vi "build waveform.vi"(10 "initialized array":dbl[][](array[numeric])) -> (2 "output waveform":waveform(dbl))   [LabVIEW 2014]
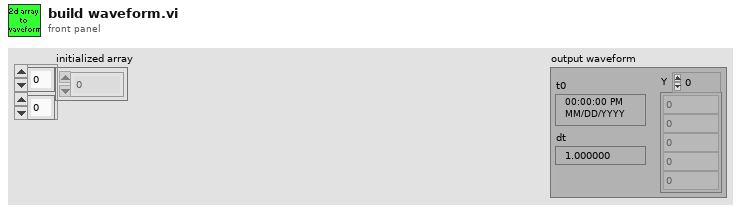
[diagram p1: front panel]
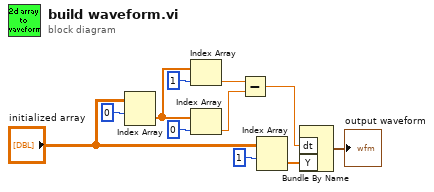
[diagram p0: block diagram]
diagram:
  n1 = Index Array(array="initialized array", index (row)=0) -> (element=w5:dbl[])  [unwired: 1 in]
  n2 = Index Array(array=w5, index=1 ("index (row)")) -> (element=w4:dbl)
  n3 = Index Array(array=w5, index=0 ("index (row)")) -> (element=w3:dbl)
  n4 = Subtract(x=w4, y=w3) -> (x-y=w2:dbl)
  n5 = Index Array(array="initialized array", index (row)=1 ("index")) -> (element=w10:dbl[])  [unwired: 1 in]
  n6 = Bundle By Name("dt"=w2, "Y"=w10) -> (→"output waveform":waveform(dbl))  [unwired: 1 in]
